vi "Obtain Broadcast Events.vi"(8 "error in":errorcluster, 10 "Create New? (F)":bool) -> (0 "error out":errorcluster, 2 "Hardware Controller Broadcast Events":T1)   [LabVIEW 2024, in "Hardware Controller.lvlib"]
doc: "This VI Obtains/Creates the Broadcast events that will be used for other modules to register to receive messages from the module that owns this VI.\n\n<b>NOTE</b>: The contents of this VI are automatically generated and modified by the <b>Tools > DQMH Consortium > DQMH</b> utilities. Consider using those utilities instead of making your own modifications to this VI.\n_____\nBased on DQMH Project Template 7.0.0.1280."
uses:
  Hardware Controller.lvlib
  Broadcast Events--cluster.ctl
  Did Init Argument--cluster.ctl
  Status Updated Argument--cluster.ctl
  Error Reported Argument--cluster.ctl
  Stop Argument--cluster.ctl
  Get Module Execution Status Argument--cluster.ctl
  System State Updated Argument--cluster.ctl
  EtherCAT Data Updated Argument--cluster.ctl
  System Fault Updated Argument--cluster.ctl
  EtherCAT Connection Status Updated Argument--cluster.ctl
  HardwareController IOLink Data Updated Argument--cluster.ctl
  IOLink Connection Updated Argument--cluster.ctl
  HardwareController EtherCAT Data Updated Argument--cluster.ctl
panel:
  # "NOTE: The contents of this VI are automatically generated and modified by the Tools > DQMH Consortium > DQMH utilities. Consider using those utilities instead of making your own modifications to this VI."
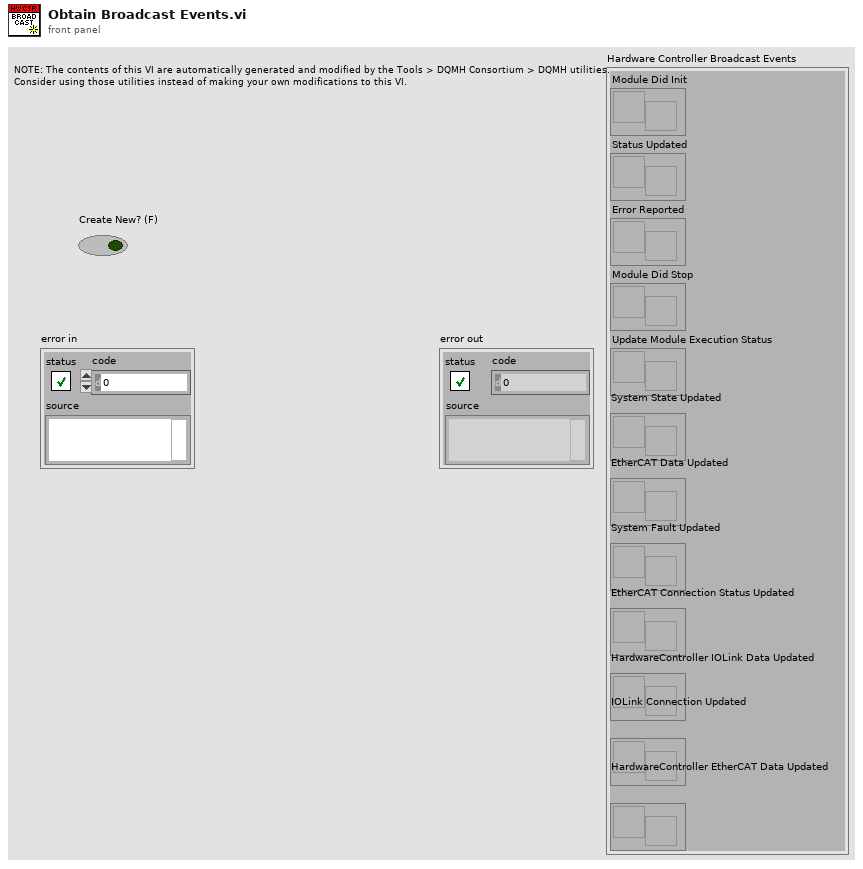
[diagram p1: front panel]
types:
  T1 = typedef "Hardware Controller.lvlib/Broadcast Events--cluster.ctl" = cluster{"Module Did Init":refnum<user-event>, "Status Updated":refnum<user-event>, "Error Reported":refnum<user-event>, "Module Did Stop":refnum<user-event>, "Update Module Execution Status":refnum<user-event>, "System State Updated":refnum<user-event>, "EtherCAT Data Updated":refnum<user-event>, "System Fault Updated":refnum<user-event>, "EtherCAT Connection Status Updated":refnum<user-event>, "HardwareController IOLink Data Updated":refnum<user-event>, "IOLink Connection Updated":refnum<user-event>, "HardwareController EtherCAT Data Updated":refnum<user-event>}
  T2 = typedef "Hardware Controller.lvlib/HardwareController EtherCAT Data Updated Argument--cluster.ctl" = cluster{"System State Out":map{string, dbl}, "System State Time":timestamp}
  T3 = typedef "Hardware Controller.lvlib/IOLink Connection Updated Argument--cluster.ctl" = cluster{"Connection State":bool}
  T4 = typedef "Hardware Controller.lvlib/HardwareController IOLink Data Updated Argument--cluster.ctl" = cluster{"System State Out":map{string, dbl}, "System State Time":timestamp}
  T5 = typedef "Hardware Controller.lvlib/EtherCAT Connection Status Updated Argument--cluster.ctl" = cluster{"EtherCAT Connection Status":bool}
  T6 = typedef "Hardware Controller.lvlib/System Fault Updated Argument--cluster.ctl" = cluster{"System Fault":bool}
  T7 = typedef "Hardware Controller.lvlib/EtherCAT Data Updated Argument--cluster.ctl" = cluster{"Process Data Input":u8[], "Process Data Output":u8[]}
  T8 = typedef "Hardware Controller.lvlib/System State Updated Argument--cluster.ctl" = cluster{"System State":map{string, dbl}}
  T9 = typedef "Hardware Controller.lvlib/Get Module Execution Status Argument--cluster.ctl" = cluster{"Running?":bool}
  T10 = typedef "Hardware Controller.lvlib/Stop Argument--cluster.ctl" = cluster{"Origin":string, "Exit via Stop Module Req?":bool, "Wait for Module to stop?":bool}
  T11 = typedef "Hardware Controller.lvlib/Error Reported Argument--cluster.ctl" = cluster{"Error":errorcluster, "Additional Information":string, "Module Name":string}
  T12 = typedef "Hardware Controller.lvlib/Status Updated Argument--cluster.ctl" = cluster{"Status":string}
  T13 = typedef "Hardware Controller.lvlib/Did Init Argument--cluster.ctl" = cluster{"Init?":bool, "Info":string}
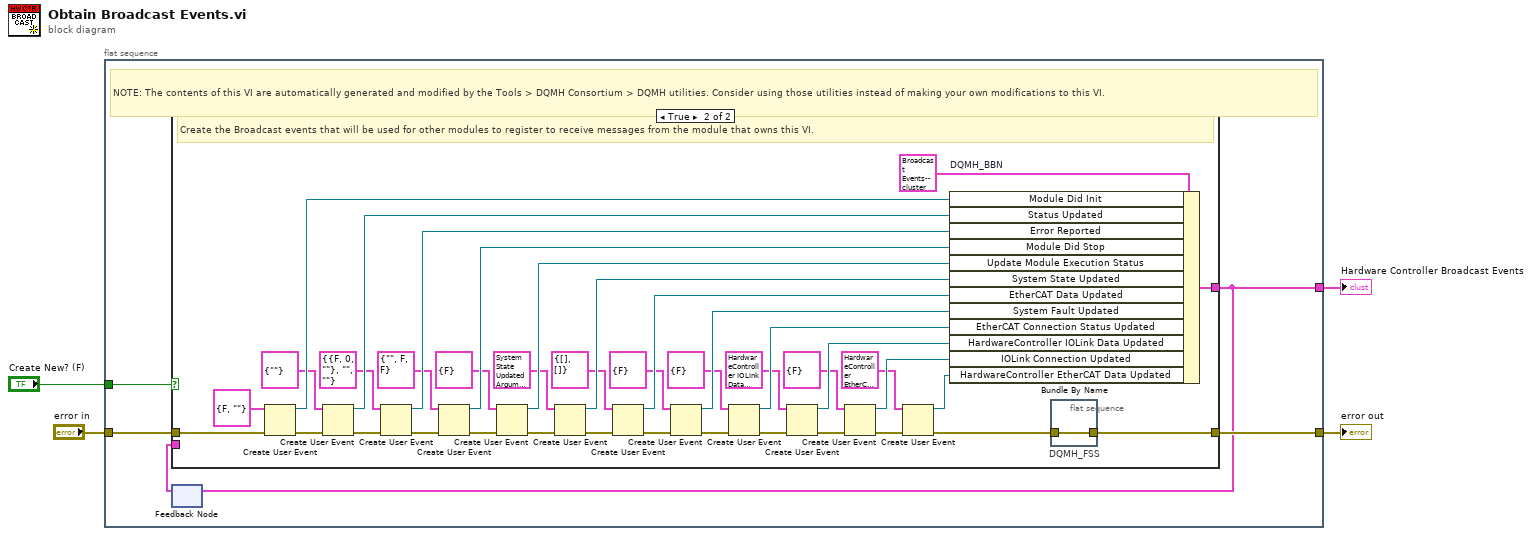
[diagram p0: block diagram]
diagram:
  n1 = flat-sequence {
    tunnel: [w9] -> w4
    tunnel: "error in" -> [w8]
    tunnel: [w6] -> w2
    tunnel: "Create New? (F)" -> [w5]
    frame #0 {
      # "NOTE: The contents of this VI are automatically generated and modified by the Tools > DQMH Consortium > DQMH utilities. Consider using those utilities instead of making your own modifications to this VI."
      n2 = feedback #1() -> (w7:T1)  [unwired: 1 in]
      n3 = case shown="True" w5 {
        tunnel: [w10 w36] -> w9
        tunnel: w8 -> [w10 w51]
        tunnel: [w11 w48] -> w6
        tunnel: w7 -> [w11 _]
        frame False {
          # "Obtain the Broadcast events that were created in a previous call to this VI."
        }
        frame True {
          # "Create the Broadcast events that will be used for other modules to register to receive messages from the module that owns this VI."
          n4 = Create User Event(user event datatype=T13 {"Init?"=FALSE, "Info"=""} ("Did Init Argument"), error in=w51) -> (user event=w49:refnum<user-event>, error out=w46:errorcluster)
          n5 = Create User Event(user event datatype=T12 {"Status"=""} ("Status Updated Argument"), error in=w46) -> (user event=w43:refnum<user-event>, error out=w45:errorcluster)
          n6 = Create User Event(user event datatype=T11 {"Error"={"status"=FALSE, "code"=0, "source"=""}, "Additional Information"="", "Module Name"=""} ("Error Reported Argument"), error in=w45) -> (user event=w40:refnum<user-event>, error out=w42:errorcluster)
          n7 = Create User Event(user event datatype=T10 {"Origin"="", "Exit via Stop Module Req?"=FALSE, "Wait for Module to stop?"=FALSE} ("Stop Argument"), error in=w42) -> (user event=w38:refnum<user-event>, error out=w37:errorcluster)
          n8 = Create User Event(user event datatype=T9 {"Running?"=FALSE} ("Get Module Execution Status Argument"), error in=w37) -> (user event=w34:refnum<user-event>, error out=w35:errorcluster)
          n9 = Create User Event(user event datatype=T8 {"System State"={}} ("System State Updated Argument"), error in=w35) -> (user event=w31:refnum<user-event>, error out=w32:errorcluster)
          n10 = Create User Event(user event datatype=T7 {"Process Data Input"=[], "Process Data Output"=[]} ("EtherCAT Data Updated Argument"), error in=w32) -> (user event=w28:refnum<user-event>, error out=w29:errorcluster)
          n11 = Create User Event(user event datatype=T6 {"System Fault"=FALSE} ("System Fault Updated Argument"), error in=w29) -> (user event=w25:refnum<user-event>, error out=w26:errorcluster)
          n12 = Create User Event(user event datatype=T5 {"EtherCAT Connection Status"=FALSE} ("EtherCAT Connection Status Updated Argument"), error in=w26) -> (user event=w22:refnum<user-event>, error out=w23:errorcluster)
          n13 = Create User Event(user event datatype=T4 {"System State Out"={}, "System State Time"=timestamp(0 s since 1904-01-01)} ("HardwareController IOLink Data Updated Argument"), error in=w23) -> (user event=w19:refnum<user-event>, error out=w20:errorcluster)
          n14 = Create User Event(user event datatype=T3 {"Connection State"=FALSE} ("IOLink Connection Updated Argument"), error in=w20) -> (user event=w16:refnum<user-event>, error out=w17:errorcluster)
          n15 = Create User Event(user event datatype=T2 {"System State Out"={}, "System State Time"=timestamp(0 s since 1904-01-01)} ("HardwareController EtherCAT Data Updated Argument"), error in=w17) -> (user event=w13:refnum<user-event>, error out=w14:errorcluster)
          n16 = Bundle By Name "DQMH_BBN"(cluster=T1 {"Module Did Init"=refnum, "Status Updated"=refnum, "Error Reported"=refnum, "Module Did Stop"=refnum, "Update Module Execution Status"=refnum, "System State Updated"=refnum, "EtherCAT Data Updated"=refnum, "System Fault Updated"=refnum, "EtherCAT Connection Status Updated"=refnum, "HardwareController IOLink Data Updated"=refnum, "IOLink Connection Updated"=refnum, "HardwareController EtherCAT Data Updated"=refnum} ("output cluster"), "Module Did Init"=w49, "Status Updated"=w43, "Error Reported"=w40, "Module Did Stop"=w38, "Update Module Execution Status"=w34, "System State Updated"=w31, "EtherCAT Data Updated"=w28, "System Fault Updated"=w25, "EtherCAT Connection Status Updated"=w22, "HardwareController IOLink Data Updated"=w19, "IOLink Connection Updated"=w16, "HardwareController EtherCAT Data Updated"=w13) -> (w48:T1)
          n17 = flat-sequence "DQMH_FSS" {
            tunnel: w14 -> [w52]
            tunnel: [w52] -> w36
            frame #0 {
            }
          }
        }
      }
      n18 = feedback-in #1(w6) -> ()
    }
  }
  "Hardware Controller Broadcast Events" <- w2
  "error out" <- w4
